vi "master_motor_mover_acceltest.vi"() -> ()   [LabVIEW 2025]
uses:
  <vilib>/ptbypt/NI_PtbyPt.lvlib
panel:
  out "Coerced Speed":dbl
  in  "Motor Speed Limit (rpm)":dbl=25.0
  in  "motor radius":dbl
  out "Speed":dbl(graph)
  out "Acceleration":dbl(graph)
  out "Known Speed (sim only)":dbl
  in  "Speed Index Selection (Sim only)":i32=1
  out "Force":dbl(graph)
  in  "stop":bool
  out "Coil A":bool
  out "Coil B":bool
  out "Coil C":bool
  out "Coil D":bool
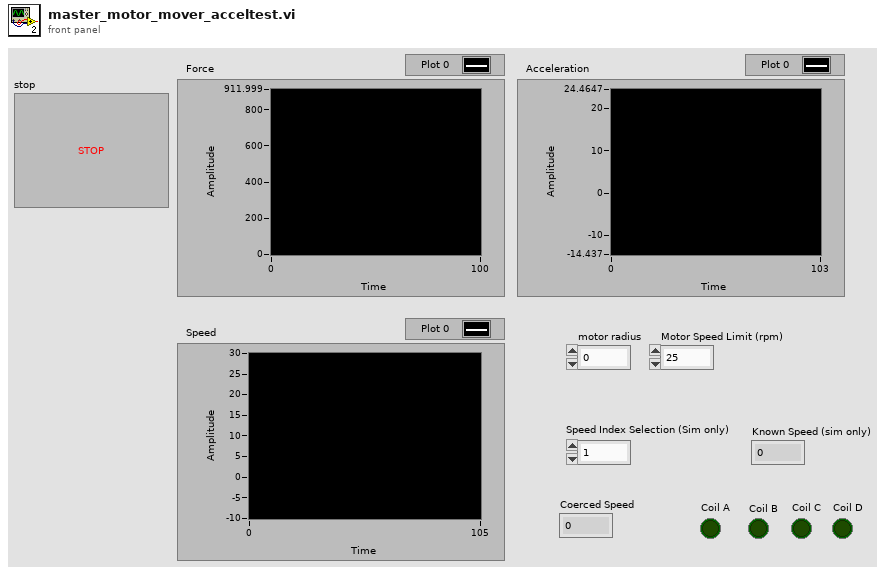
[diagram p1: front panel]
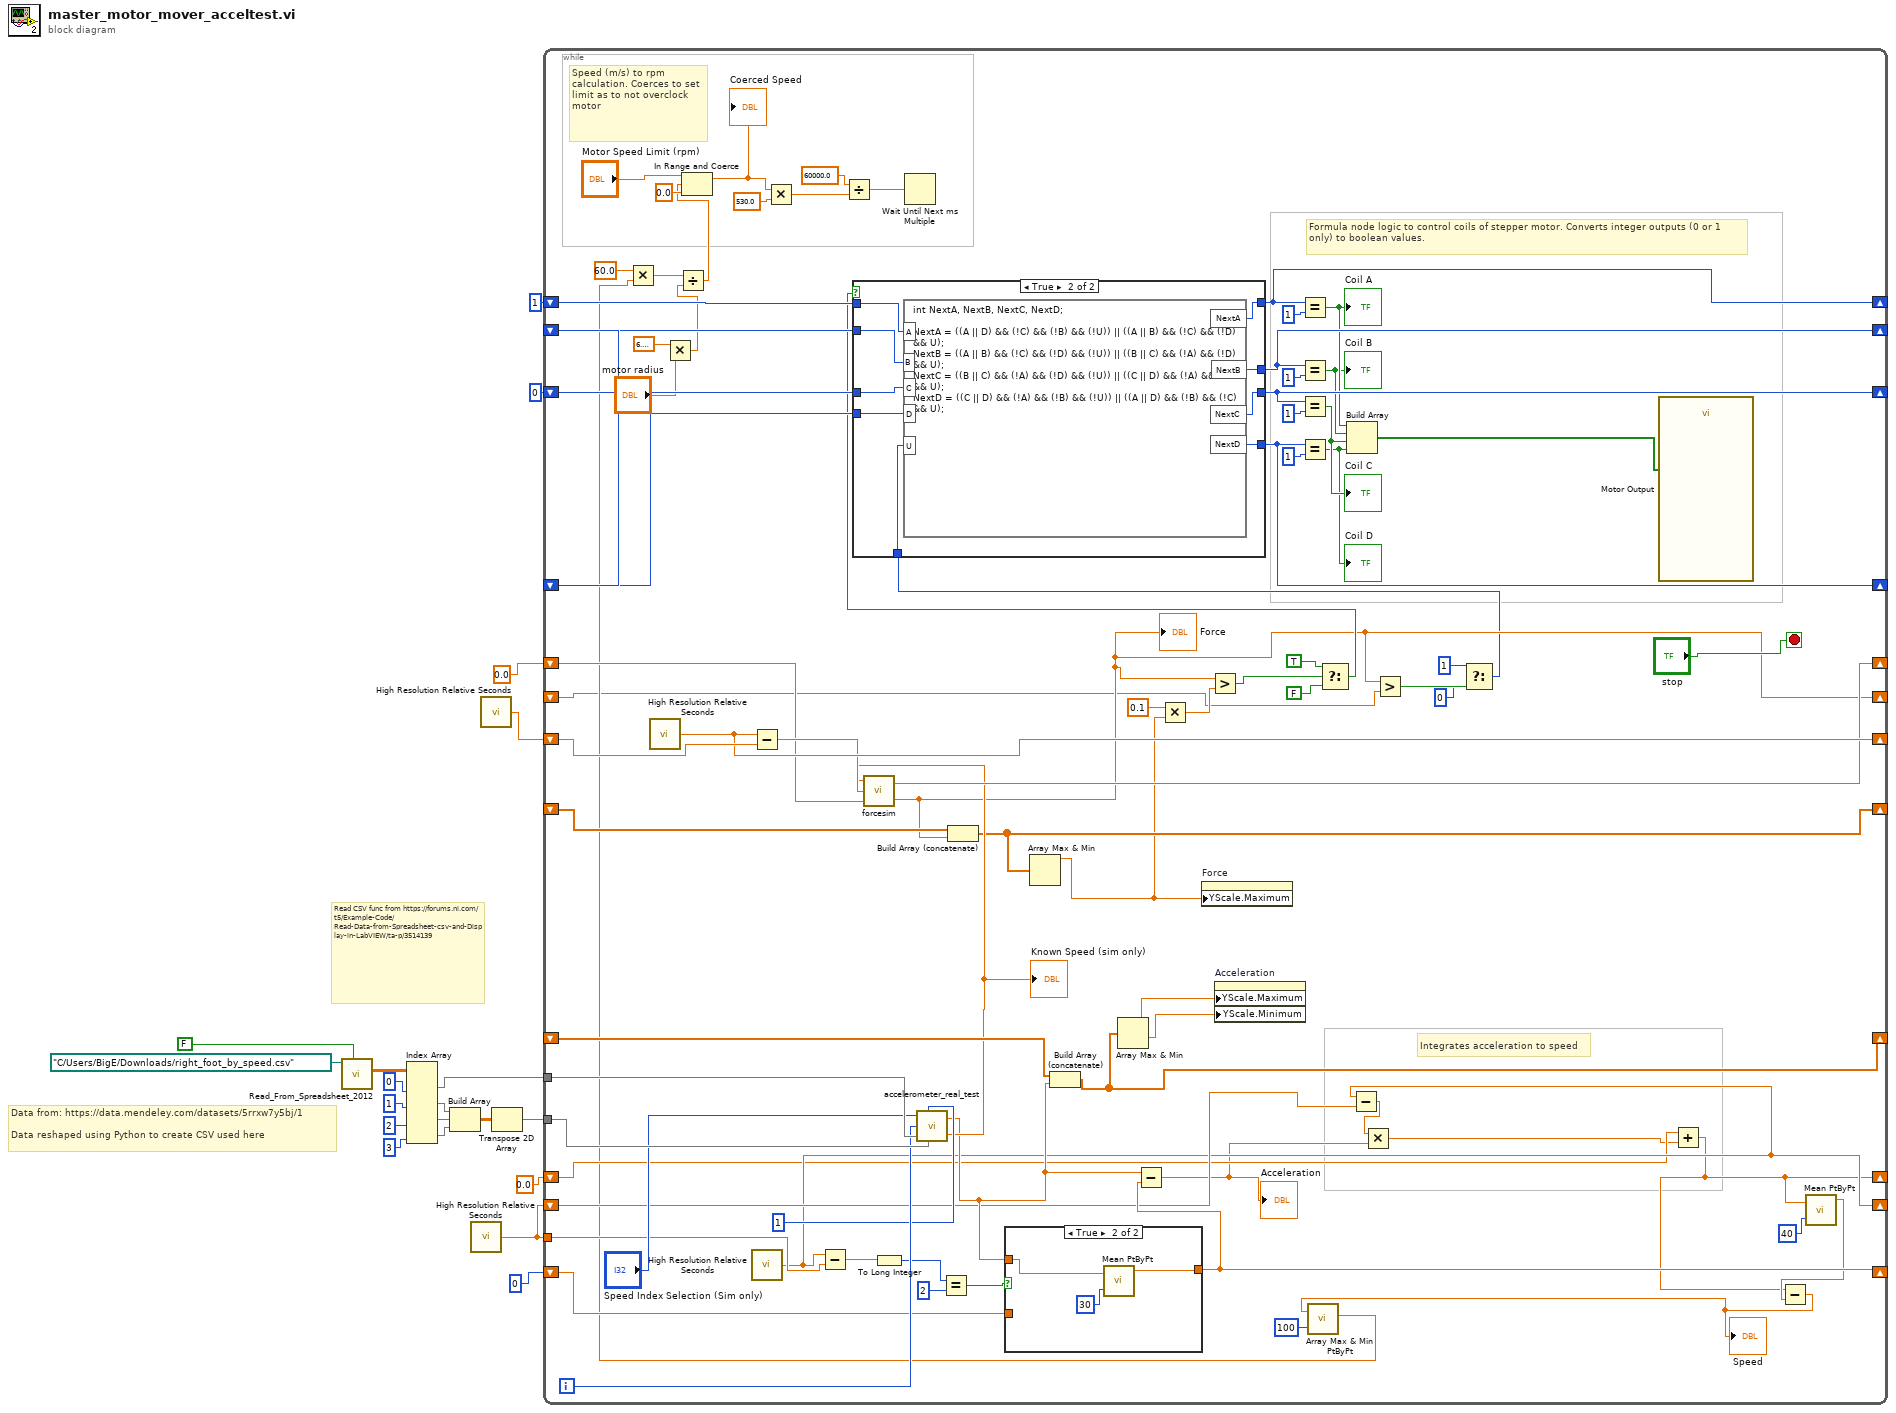
[diagram p0: block diagram]
diagram:
  w19 = 0
  # "Data from: https://data.mendeley.com/datasets/5rrxw7y5bj/1\n\nData reshaped using Python to create CSV used here"
  # "Read CSV func from https://forums.ni.com/t5/Example-Code/Read-Data-from-Spreadsheet-csv-and-Display-in-LabVIEW/ta-p/3514139"
  n1 = call "Read_From_Spreadsheet_2012.vi"("My File has Row Headers"=FALSE, "Spreadsheet path (.csv)"=path "C:/Users/BigE/Downloads/right_foot_by_speed.csv") -> ("Data Dsiplay"=w12:dbl[][])  [unwired: 8 in, 1 out]
  n2 = Index Array(array=w12, index (col) #1=0 ("disabled index (col)"), index (col) #2=1 ("disabled index (col)"), index (col) #3=2 ("disabled index (col)"), index (col) #4=3 ("disabled index (col)")) -> (element #1=w5:dbl[], element #2=w13:dbl[], element #3=w14:dbl[], element #4=w15:dbl[])  [unwired: 4 in]
  n3 = Build Array(w13, w14, w15) -> (w16:dbl[][])
  n4 = call <vilib>:"High Resolution Relative Seconds.vi"() -> ("relative seconds"=w2:dbl)
  n5 = call <vilib>:"High Resolution Relative Seconds.vi"() -> ("relative seconds"=w17:dbl)
  n6 = Transpose 2D Array(2D array=w16) -> (transposed array=w4:dbl[][])
  n7 = while {
    shift-right: [w90] -> _
    shift-left: 1 -> [w94]
    shift-right: [w89] -> _
    shift-left: w19 -> [w93]
    shift-right: [w88] -> _
    shift-left: w19 -> [w92]
    shift-right: [w87] -> _
    shift-left: w19 -> [w91]
    shift-right: [w75] -> _
    shift-left: 0.0 -> [w76]
    shift-right: [w78] -> _
    shift-left: w17 -> [w79]
    tunnel: w5 -> [w73]
    tunnel: w4 -> [w72]
    shift-right: [w34] -> _
    shift-left: _ -> [w74]
    shift-right: [w67] -> _
    shift-left: _ -> [w68]
    shift-right: [w61] -> _
    shift-left: 0 ("x,y,z? 2") -> [w63]
    tunnel: w2 -> [w58]
    shift-right: [w54] -> _
    shift-left: w2 -> [w55]
    shift-right: [w47] -> _
    shift-left: 0.0 ("x") -> [w52]
    shift-right: [w26] -> _
    shift-left: _ -> [w25]
    i -> [w71]
    stop <- "stop" stop-if-true
    # "Integrates acceleration to speed"
    # "Formula node logic to control coils of stepper motor. Converts integer outputs (0 or 1 only) to boolean values."
    # "Speed (m/s) to rpm calculation. Coerces to set limit as to not overclock motor"
    n8 = call <vilib>:"High Resolution Relative Seconds.vi"() -> ("relative seconds"=w78:dbl)
    n9 = Multiply(x=6.283185307179586, y="motor radius") -> (x*y=w39:dbl)
    n10 = Subtract(x=w78, y=w79) -> (x-y=w77:dbl)
    n11 = call <vilib>:"High Resolution Relative Seconds.vi"() -> ("relative seconds"=w54:dbl)
    n12 = Subtract(x=w54, y=w58) -> (x-y=w57:dbl)
    n13 = To Long Integer(number=w57) -> (32bit integer=w56:i32)
    n14 = call "accelerometer_real_test.vi"("Speed Index"="Speed Index Selection (Sim only)", "x,y,z?"=1 ("x,y,z? 2"), "i"=w71, "speed subarray"=w73, "transposed array"=w72) -> ("Acceleration"=w62:dbl, "Speed"=w64:dbl)
    "Known Speed (sim only)" <- w64
    n15 = call "forcesim.vi"("Phase"=w76, "dT"=w77, "Speed"=w64) -> ("Force"=w26:dbl, "Phase Out"=w75:dbl)
    "Force" <- w26
    n16 = Equal?(x=w56, y=2) -> (x = y?=w60:bool)
    n17 = Build Array (concatenate)(w74, w26) -> (w34:dbl[])
    n18 = case shown="True" w60 {
      tunnel: w62 -> [_ w104]
      tunnel: [w102 w103] -> w61
      tunnel: w63 -> [w102 _]
      frame False {
      }
      frame True {
        n19 = call <vilib>:"Mean PtByPt.vi"("x"=w104, "sample length"=30) -> ("mean"=w103:dbl)  [unwired: 2 in, 1 out]
      }
    }
    n20 = Array Max & Min(array=w34) -> (max value=w32:dbl)  [unwired: 3 out]
    n21 = Build Array (concatenate)(w68, w62) -> (w67:dbl[])
    n22 = Array Max & Min(array=w67) -> (max value=w65:dbl, min value=w66:dbl)  [unwired: 2 out]
    n23 = Subtract(x=w62, y=w61) -> (x-y=w51:dbl)
    "Acceleration" <- w51
    n24 = Multiply(x=0.1, y=w32) -> (x*y=w31:dbl)
    n25 = property on="Force" class="WFChart (strict)"("YScale.Maximum"=w32) -> ()  [unwired: 2 in, 2 out]
    n26 = Greater?(x=w26, y=w31) -> (0:w30:bool)
    n27 = property on="Acceleration" class="WFChart (strict)"("YScale.Maximum"=w65, "YScale.Minimum"=w66) -> ()  [unwired: 2 in, 2 out]
    n28 = Select(t=TRUE, s=w30, f=FALSE) -> (s? t:f=w27:bool)
    n29 = Subtract(x=w54, y=w55) -> (x-y=w53:dbl)
    n30 = Multiply(x=w53, y=w51) -> (x*y=w50:dbl)
    n31 = Greater?(x=w26, y=w25) -> (0:w24:bool)
    n32 = Select(t=1, s=w24, f=0) -> (s? t:f=w21:i32)
    n33 = case shown="True" w27 {
      tunnel: w94 -> [w109 w115]
      tunnel: w93 -> [w108 w116]
      tunnel: w92 -> [w107 w118]
      tunnel: w91 -> [w106 w117]
      tunnel: [w109 w114] -> w90
      tunnel: [w108 w113] -> w89
      tunnel: [w107 w112] -> w88
      tunnel: [w106 w111] -> w87
      tunnel: w21 -> [_ w110]
      frame False {
      }
      frame True {
        n34 = formula code="int NextA, NextB, NextC, NextD;\n\nNextA = ((A || D) && (!C) && (!B) && (!U)) || ((A || B) && (!C) && (!D) && U);\nNextB = ((A || B) && (!C) && (!D) && (!U)) || ((B || C) && (!A) && (!D) && U);\nNextC = ((B || C) && (!A) && (!D) && (!U)) || ((C || D) && (!A) && (!B) && U);\nNextD = ((C || D) && (!A) && (!B) && (!U)) || ((A || D) && (!B) && (!C) && U);"("A"=w115, "B"=w116, "C"=w118, "D"=w117, "U"=w110) -> ("NextA"=w114:i32, "NextB"=w113:i32, "NextC"=w112:i32, "NextD"=w111:i32)
      }
    }
    n35 = Equal?(x=w90, y=1) -> (x = y?=w85:bool)
    "Coil A" <- w85
    n36 = Equal?(x=w89, y=1) -> (x = y?=w84:bool)
    "Coil B" <- w84
    n37 = Equal?(x=w88, y=1) -> (x = y?=w83:bool)
    "Coil C" <- w83
    n38 = Equal?(x=w87, y=1) -> (x = y?=w82:bool)
    "Coil D" <- w82
    n39 = Build Array(w85, w84, w83, w82) -> (w81:bool[])
    n40 = call "Motor Output"("data"=w81) -> ()  [unwired: 17 in, 2 out]
    n41 = Add(x=w52, y=w50) -> (x+y=w47:dbl)
    n42 = call <vilib>:"Mean PtByPt.vi"("x"=w47, "sample length"=40) -> ("mean"=w48:dbl)  [unwired: 2 in, 1 out]
    n43 = Subtract(x=w47, y=w48) -> (x-y=w45:dbl)
    "Speed" <- w45
    n44 = call <vilib>:"Array Max & Min PtByPt.vi"("input data point"=w45, "sample length"=100) -> ("max value"=w43:dbl)  [unwired: 1 in, 4 out]
    n45 = Multiply(x=60.0, y=w43) -> (x*y=w42:dbl)
    n46 = Divide(x=w42, y=w39) -> (x/y=w36:dbl)
    n47 = In Range and Coerce(upper limit="Motor Speed Limit (rpm)", x=w36, lower limit=0.0) -> (coerced(x)=w35:dbl)  [unwired: 1 out]
    "Coerced Speed" <- w35
    n48 = Multiply(x=w35, y=530.0) -> (x*y=w97:dbl)
    n49 = Divide(x=60000.0, y=w97) -> (x/y=w86:dbl)
    n50 = Wait Until Next ms Multiple(millisecond multiple=w86) -> ()  [unwired: 1 out]
  }
